vi "deploy alarm map.vi"() -> ()   [LabVIEW 2016, in "Alarm interface.lvlib"]
uses:
  Alarm interface.lvlib
panel:
  in  "导入":bool
  in  "导出":bool
  in  "Project":i32(listbox)
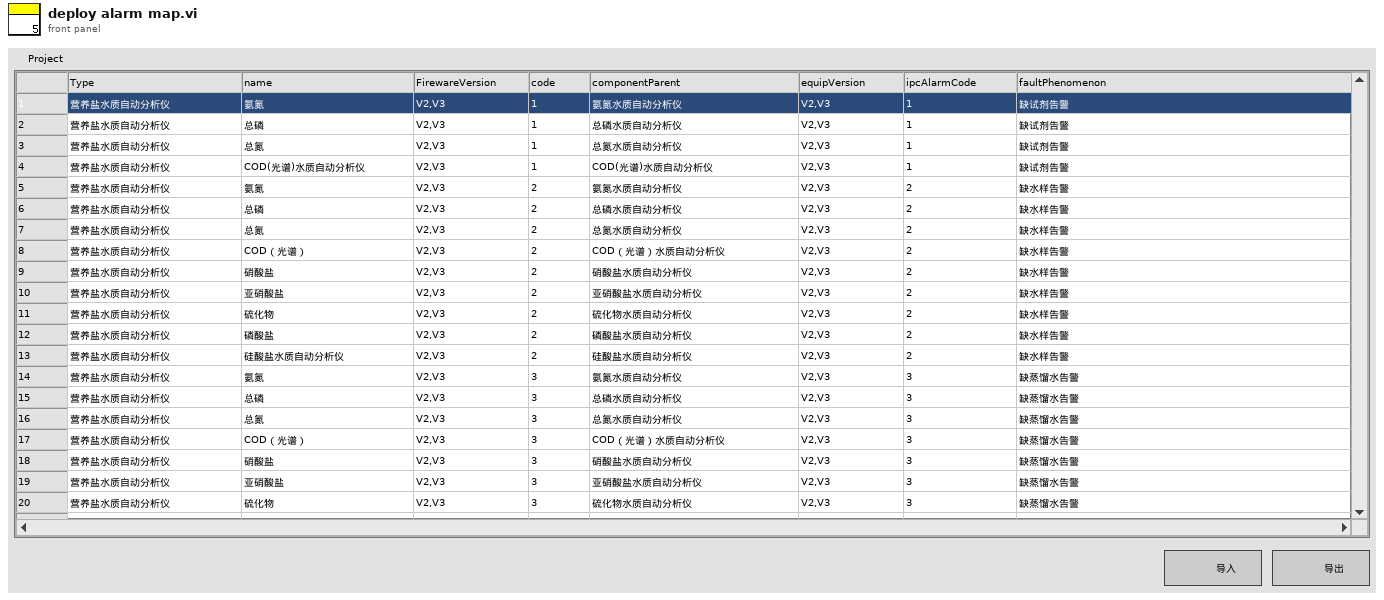
[diagram p1: front panel]
types:
  T1 = typedef "Alarm interface.lvlib/map project.ctl" = cluster{"data":T2[]}
  T2 = typedef "Alarm interface.lvlib/map data.ctl" = cluster{"map in":T3, "map out":T4}
  T3 = typedef "Alarm interface.lvlib/map in.ctl" = cluster{"name":string, "FirmwareVersion":string, "code":string}
  T4 = typedef "Alarm interface.lvlib/map out.ctl" = cluster{"componentParent":string, "equipVersion":string, "ipcAlarmCode":string, "faultPhenomenon":string}
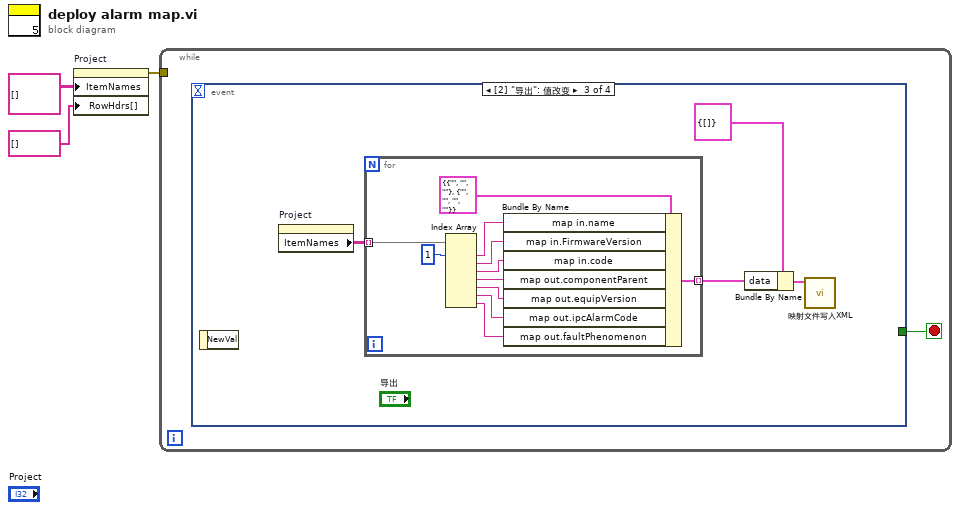
[diagram p0: block diagram]
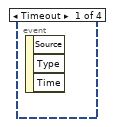
[diagram p2: hidden frame]
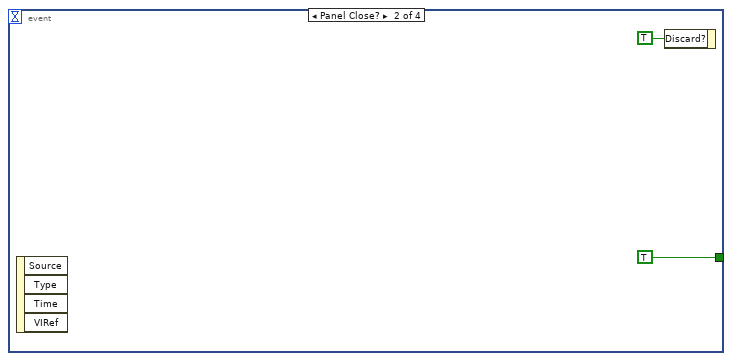
[diagram p3: hidden frame]
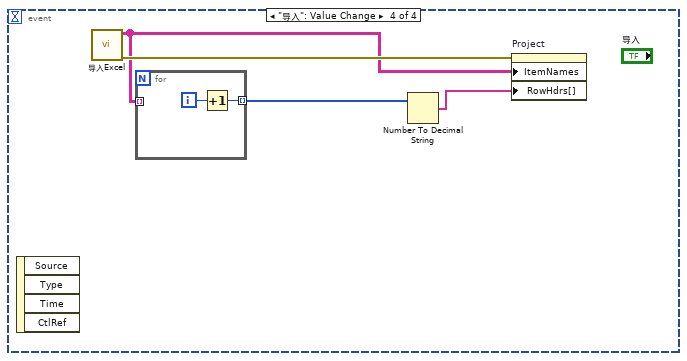
[diagram p4: hidden frame]
diagram:
  n1 = property on="Project" class="MCListbox (严格)"("ItemNames"=string[][] [] ("项名"), "RowHdrs[]"=string[] [] ("行首字符串[]")) -> (error out=w1:errorcluster)  [unwired: 2 in, 1 out]
  n2 = while {
    tunnel: w1 -> [_]
    stop <- w4 stop-if-true
    n3 = event shown="[2] \"导出\": 值改变" {
      selector: _ -> [_ _ _ _]
      dyn-events: _ -> [_ _ _ _]
      timeout: _ -> [_ _ _ _]
      tunnel: [_ TRUE _ _] -> w4
      event Timeout {
        n4 = event-data() -> ()  [unwired: 1 in, 3 out]
      }
      event Panel Close? {
        n5 = event-data() -> ()  [unwired: 1 in, 4 out]
        n6 = event-data("Discard?"=TRUE ("放弃？")) -> ()  [unwired: 1 in, 1 out]
      }
      event "导出": Value Change {
        n7 = event-data() -> ()  [unwired: 1 in, 1 out]
        n8 = property on="Project" class="MCListbox (严格)"() -> ("ItemNames"=w10:string[][])  [unwired: 2 in, 2 out]
        n9 = for {
          tunnel: w10 -> [w21] mode=indexing
          tunnel: [w12] -> w8 mode=indexing
          n10 = Index Array(array=w21, index #1=1 ("索引")) -> (element #1=w19:string, element #2=w18:string, element #3=w13:string, element #4=w17:string, element #5=w16:string, element #6=w15:string, element #7=w14:string)  [unwired: 6 in]
          n11 = Bundle By Name(cluster=T2 {"map in"={"name"="", "FirmwareVersion"="", "code"=""}, "map out"={"componentParent"="", "equipVersion"="", "ipcAlarmCode"="", "faultPhenomenon"=""}} ("data"), "map in.name"=w19, "map in.FirmwareVersion"=w18, "map in.code"=w13, "map out.componentParent"=w17, "map out.equipVersion"=w16, "map out.ipcAlarmCode"=w15, "map out.faultPhenomenon"=w14) -> (w12:T2)
        }
        n12 = Bundle By Name(cluster=T1 {"data"=[]} ("Project"), "data"=w8) -> (w7:T1)
        n13 = call "映射文件写入XML.vi"("project"=w7) -> ()  [unwired: 10 in, 1 out]
      }
      event "导入": Value Change {
        n14 = event-data() -> ()  [unwired: 1 in, 4 out]
        n15 = call "导入Excel.vi"() -> ("error out"=w25:errorcluster, "data"=w24:string[][])  [unwired: 10 in]
        n16 = for {
          tunnel: w24 -> [_] mode=indexing
          tunnel: [w26] -> w23 mode=indexing
          i -> [w27]
          n17 = Increment(x=w27) -> (x+1=w26:i32)
        }
        n18 = Number To Decimal String(number=w23) -> (decimal integer string=w22:string[])  [unwired: 1 in]
        n19 = property on="Project" class="MCListbox (严格)"(error in=w25, "ItemNames"=w24, "RowHdrs[]"=w22) -> ()  [unwired: 1 in, 2 out]
      }
    }
  }
